vi "Func-칼만 필터.vi"(3 "프런트패널 윈도우:모니터":u16) -> ()   [LabVIEW 2015]
panel:
  in  "Interval time(ms)":u32
  in  "x set":dbl(slide) step=1.0 scale=0.0..5.0 scale format="%#_6f"
  in  "Exit":bool
  out "Ready":bool
  out "Numeric Control":i32
  out "Drawing Time(ms)":u32=10
  in  "R":dbl=0.9999999999999999 min=0.0 max=1000.0 step=0.1 format="%#.3f"
  in  "Q":dbl=0.05 min=0.0 max=1000.0 step=0.01 format="%#.3f"
  out "그래프":cluster{"x":dbl, "z":dbl}(graph)
  out "Kalman X":dbl=759.7992239190703 format="%.5f"
  out "Real X":dbl=735.0 format="%.5f"
  # "시뮬레이션 - 칼만 필터"
  # "필터 게인 설정"
  # "Q: 예측 노이즈 공분산\n    값이 작을수록 무겁게 동작\nR: 측정 노이즈 공분산\n    값이 클수록 무겁게 동작"
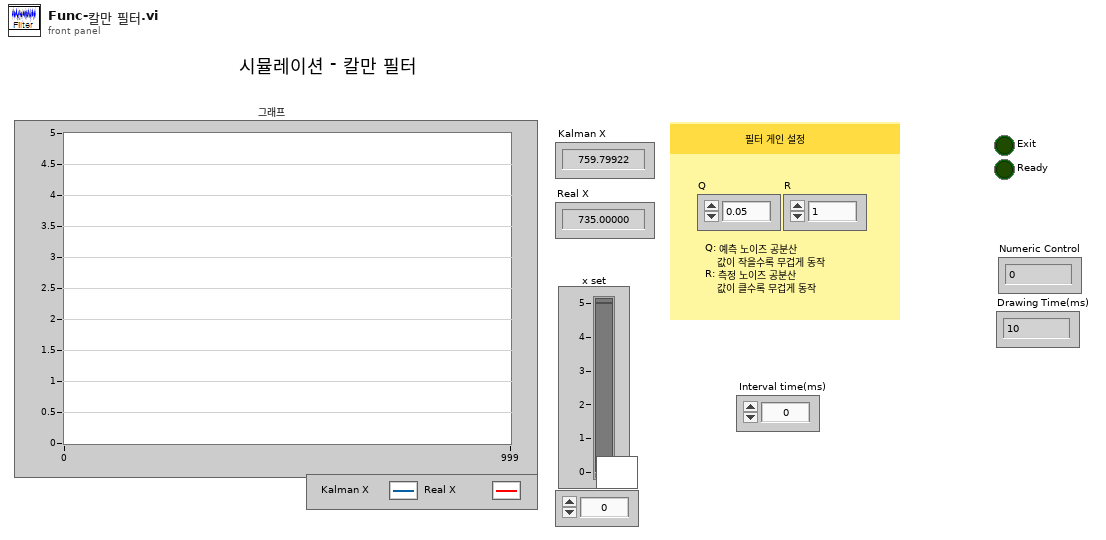
[diagram p1: front panel]
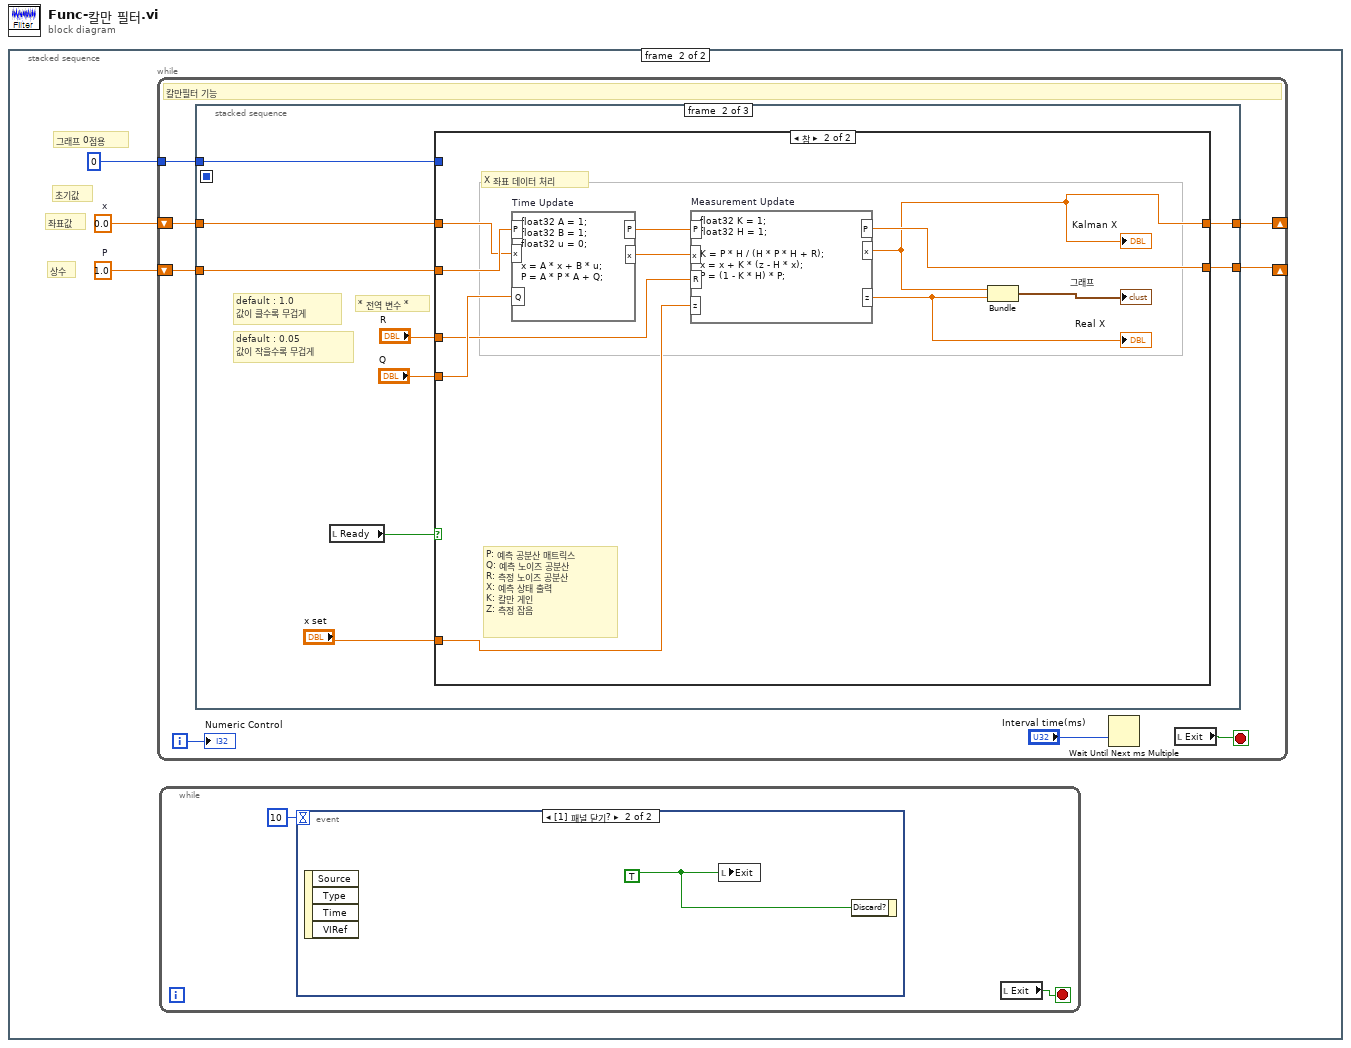
[diagram p0: block diagram]
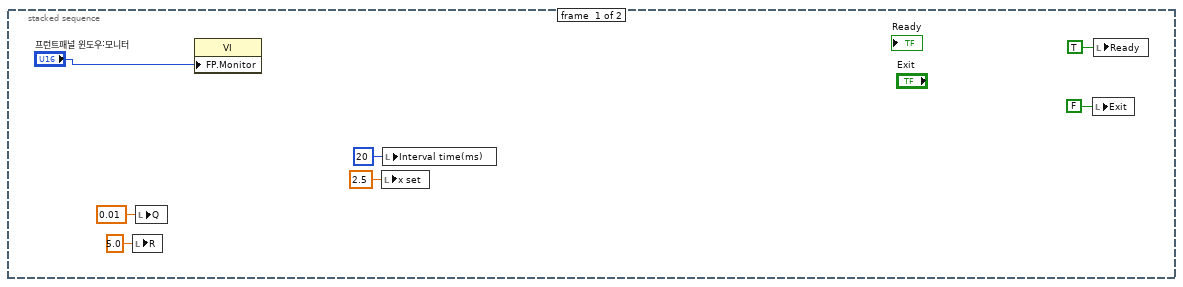
[diagram p2: hidden frame]
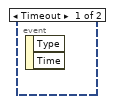
[diagram p3: hidden frame]
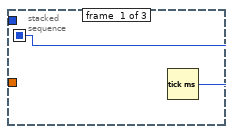
[diagram p4: hidden frame]
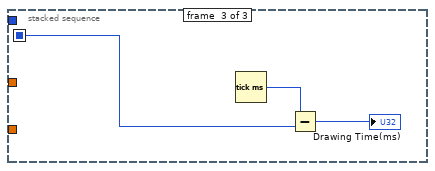
[diagram p6: hidden frame]
diagram:
  n1 = stacked-sequence {
    frame #0 {
      n2 = local write "R"(5.0 ("R")) -> ()
      n3 = local write "Q"(0.01 ("Q")) -> ()
      n4 = property class="VI"("FP.Monitor"="프런트패널 윈도우:모니터") -> ()  [unwired: 2 in, 2 out]
      n5 = local write "x set"(2.5 ("x set")) -> ()
      n6 = local write "Interval time(ms)"(u32 20 ("Interval time(ms)")) -> ()
      n7 = local write "Exit"(FALSE ("Exit")) -> ()
      n8 = local write "Ready"(TRUE ("Ready")) -> ()
    }
    frame #1 {
      w8 = 1.0  # P
      w9 = 0.0  # x
      # "좌표값"
      # "상수"
      # "초기값"
      # "그래프 0점용"
      n9 = while {
        shift-right: [w17] -> _
        shift-left: w9 -> [w20]
        shift-right: [w19] -> _
        shift-left: w8 -> [w21]
        tunnel: 0 -> [w18]
        i -> [w16]
        stop <- w15 stop-if-true
        # "칼만필터 기능"
        n10 = stacked-sequence {
          seq-local: [w22 _ _] -> [_ _ w46]
          tunnel: w21 -> [_ w25 _]
          tunnel: w20 -> [_ w31 _]
          tunnel: [_ w30 _] -> w19
          tunnel: w18 -> [_ w29 _]
          tunnel: [_ w28 _] -> w17
          frame #0 {
            n11 = Tick Count (ms)() -> (millisecond timer value=w22:u32)
          }
          frame #1 {
            # "* 전역 변수 *"
            # "default : 0.05\n값이 작을수록 무겁게"
            # "default : 1.0\n값이 클수록 무겁게"
            n12 = local read "Ready"() -> (w24:bool)
            n13 = case shown="참" w24 {
              tunnel: w25 -> [w32 w44]
              tunnel: w31 -> [w33 w41]
              tunnel: [w32 w40] -> w30
              tunnel: w29 -> [_ _]
              tunnel: [w33 w34] -> w28
              tunnel: "Q" -> [_ w37]
              tunnel: "R" -> [_ w36]
              tunnel: "x set" -> [_ w35]
              frame False {
              }
              frame True {
                # "P: 예측 공분산 매트릭스\nQ: 예측 노이즈 공분산\nR: 측정 노이즈 공분산\nX: 예측 상태 출력 \nK: 칼만 게인\nZ: 측정 잡음"
                # "X 좌표 데이터 처리"
                n14 = formula code="float32 A = 1;\nfloat32 B = 1;\nfloat32 u = 0;\n\nx = A * x + B * u;\nP = A * P * A + Q;" "Time Update"("x"=w41, "P"=w44, "Q"=w37) -> ("x"=w43:dbl, "P"=w42:dbl)
                n15 = formula code="float32 K = 1;\nfloat32 H = 1;\n\nK = P * H / (H * P * H + R);\nx = x + K * (z - H * x);\nP = (1 - K * H) * P;" "Measurement Update"("x"=w43, "P"=w42, "z"=w35, "R"=w36) -> ("x"=w34:dbl, "P"=w40:dbl, "z"=w38:dbl)
                "Kalman X" <- w34
                "Real X" <- w38
                n16 = Bundle("x"=w34, "z"=w38) -> (→"그래프":cluster{"x":dbl, "z":dbl})  [unwired: 1 in]
              }
            }
          }
          frame #2 {
            n17 = Tick Count (ms)() -> (millisecond timer value=w47:u32)
            n18 = Subtract(x=w47, y=w46) -> (x-y=→"Drawing Time(ms)":u32)
          }
        }
        n19 = Wait Until Next ms Multiple(millisecond multiple="Interval time(ms)") -> ()  [unwired: 1 out]
        n20 = local read "Exit"() -> (w15:bool)
        "Numeric Control" <- w16
      }
      n21 = while {
        stop <- w11 stop-if-true
        n22 = event shown="[1] 패널 닫기?" {
          selector: _ -> [_ _]
          dyn-events: _ -> [_ _]
          timeout: 10 -> [_ _]
          event Timeout {
            n23 = event-data() -> ()  [unwired: 1 in, 2 out]
          }
          event Panel Close? {
            w13 = TRUE ("Exit")
            n24 = event-data() -> ()  [unwired: 1 in, 4 out]
            n25 = local write "Exit"(w13) -> ()
            n26 = event-data("Discard?"=w13) -> ()  [unwired: 1 in, 1 out]
          }
        }
        n27 = local read "Exit"() -> (w11:bool)
      }
    }
  }
